vi "Begin.vi"(11 "Image Size":T1=enum."160x120") -> (0 "error out":errorcluster)   [LabVIEW 2011]
doc: "Called before other user functions, this VI is expected to open initial I/O refnums, load in file data, and do all program initialization. Notice that the <B>error out</B> terminal is simply used for data flow. Wiring it to other structures or subVIs ensures that this VI runs first."
uses:
  <vilib>/Rock Robotics/WPI/Camera/WPI_CameraImageSize.ctl
  <vilib>/Rock Robotics/SystemInterfaces/DIO/FPGA_DIOPWMChannel.ctl
  <vilib>/Rock Robotics/WPI/Joystick/WPI_JoystickDeviceEnum.ctl
  <vilib>/Rock Robotics/WPI/Camera/WPI_CameraWhite Balance Values.ctl
  <vilib>/Rock Robotics/WPI/Camera/WPI_CameraExposure Values.ctl
  <vilib>/Rock Robotics/WPI/Camera/WPI_CameraFrameRate.ctl
  <vilib>/Rock Robotics/SystemInterfaces/DIO/FPGA_DIOChannel.ctl
  <vilib>/Rock Robotics/WPI/Solenoid/WPI_SolenoidChannel.ctl
  <vilib>/Rock Robotics/SystemInterfaces/DIO/FPGA_DIORelayChannel.ctl
  <vilib>/Rock Robotics/SystemInterfaces/AI/FPGA_AIGyroChannel.ctl
  <vilib>/Rock Robotics/SystemInterfaces/Typedef/FPGA_TypedefDigitalModule.ctl
  <vilib>/Rock Robotics/WPI/Solenoid/WPI_SolenoidValue.ctl
  <vilib>/Rock Robotics/WPI/RobotDrive/WPI_RobotDriveOpen4MotorWithJaguar.vi
  <vilib>/Rock Robotics/WPI/Solenoid/WPI_SolenoidOpenDouble.vi
  <vilib>/Rock Robotics/WPI/Counter/WPI_CounterDigitalInputToDigitalSource.vi
  <vilib>/Rock Robotics/WPI/Counter/WPI_CounterOpen Gear Tooth Sensor Mode.vi
  <vilib>/Rock Robotics/WPI/MotorControl/WPI_MotorControlOpen Jaguar.vi
  <vilib>/Rock Robotics/WPI/Solenoid/WPI_SolenoidOpenSingle.vi
  <vilib>/Rock Robotics/WPI/Solenoid/WPI_SolenoidSetEnum.vi
  <vilib>/Rock Robotics/WPI/Counter/WPI_CounterOpen Semi Period Mode.vi
  <vilib>/Rock Robotics/WPI/MotorControl/WPI_MotorControlOpen Victor.vi
  <vilib>/Rock Robotics/WPI/Compressor/WPI_CompressorGetSetRefNum.vi
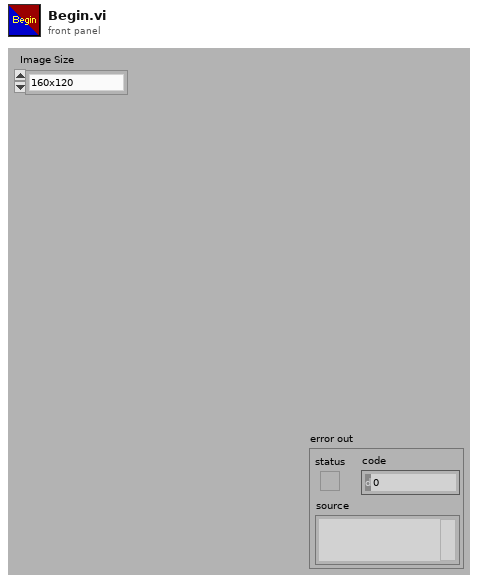
[diagram p1: front panel]
types:
  T1 = typedef "WPI_CameraImageSize.ctl" = enum16{"640x480", "320x240", "160x120"}
  T2 = typedef "FPGA_DIOPWMChannel.ctl" = enum8{"PWM 1", "PWM 2", "PWM 3", "PWM 4", "PWM 5", "PWM 6", "PWM 7", "PWM 8", "PWM 9", "PWM 10", "Invalid"}
  T3 = typedef "FPGA_DIOChannel.ctl" = enum8{"DIO 1", "DIO 2", "DIO 3", "DIO 4", "DIO 5", "DIO 6", "DIO 7", "DIO 8", "DIO 9", "DIO 10", "DIO 11", "DIO 12", "DIO 13", "DIO 14", "Invalid"}
  T4 = typedef "WPI_SolenoidValue.ctl" = enum16{"Off", "On", "Forward", "Reverse"}
  T5 = typedef "WPI_SolenoidChannel.ctl" = enum8{"Solenoid 1", "Solenoid 2", "Solenoid 3", "Solenoid 4", "Solenoid 5", "Solenoid 6", "Solenoid 7", "Solenoid 8", "Invalid"}
  T6 = typedef "WPI_JoystickDeviceEnum.ctl" = enum16{"USB 1", "USB 2", "USB 3", "USB 4", "Kinect 1", "Kinect 2"}
  T7 = typedef "FPGA_TypedefDigitalModule.ctl" = enum16{"Digital Module 1", "Digital Module 2"}
  T8 = typedef "FPGA_AIGyroChannel.ctl" = enum8{"AI 1", "AI 2", "Invalid"}
  T9 = typedef "FPGA_DIORelayChannel.ctl" = enum8{"Relay 1", "Relay 2", "Relay 3", "Relay 4", "Relay 5", "Relay 6", "Relay 7", "Relay 8", "Invalid"}
  T10 = typedef "WPI_CameraFrameRate.ctl" = u32
  T11 = typedef "WPI_CameraExposure Values.ctl" = enum16{"Auto", "Flicker-free 50 Hz", "Flicker-free 60 Hz", "Hold current"}
  T12 = typedef "WPI_CameraWhite Balance Values.ctl" = enum16{"Auto", "Fixed indoor", "Fixed outdoor 1", "Fixed outdoor 2", "Fixed fluorescent 1", "Fixed fluorescent 2", "Hold current"}
  T13 = typedef "WPI_RobotDriveDevRef.ctl" = cluster{"DevStatus":errorcluster, "Motors[]":T14[], "Square Inputs":bool, "Max Output":dbl, "Isochronous":bool}
  T14 = typedef "WPI_MotorControlDeviceRef.ctl" = cluster{"DeviceStatus":errorcluster, "Type":enum16{"PWM", "CAN"}, "PWM":cluster{"Digital Module":T7, "PWM Channel":T2, "DeadBand":T15}, "CAN":cluster{"Device Number":u8, "Control Mode":T16, "Semaphore":T17, "Max Vout":dbl}, "Invert":bool, "TransformRef":T18, "InvTransformRef":T18}
  T15 = typedef "WPI_PWMDeadband.ctl" = cluster{"Name":string, "maxPositivePwm":i32, "minPositivePwm":i32, "centerPwm":i32, "maxNegativePwm":i32, "minNegativePwm":i32, "angularRange":u16}
  T16 = typedef "WPI_CANJaguar_ControlMode.ctl" = enum8{"Percent VBus", "Current", "Speed", "Position", "Voltage"}
  T17 = typedef "Semaphore RefNum" = refnum<k1>
  T18 = typedef "WPI_PWMTransform_ConPane.ctl" = refnum<vi>
  T19 = typedef "WPI_JoystickDevRef.ctl" = cluster{"Device":T6}
  T20 = typedef "WPI_DigitalInputDevRef.ctl" = cluster{"DevStatus":errorcluster, "DIO Channel":T3, "Digital Module":T7}
  T21 = typedef "WPI_SolenoidDevRef.ctl" = cluster{"DevStatus":errorcluster, "Solenoid Module":T22, "Forward Solenoid Channel":T5, "Reverse Solenoid Channel":T5}
  T22 = typedef "FPGA_TypedefSolenoidModule.ctl" = enum16{"Solenoid Module 1", "Solenoid Module 2"}
  T23 = typedef "WPI_GyroDevRef.ctl" = cluster{"DevStatus":errorcluster, "Analog Module":T24, "Analog Channel":T25, "Offset":dbl, "Gain (VoltsPerDegree/Second)":dbl}
  T24 = typedef "FPGA_TypedefAnalogModule.ctl" = enum16{"Analog Module 1", "Analog Module 2"}
  T25 = typedef "FPGA_AIChannel.ctl" = enum8{"AI 1", "AI 2", "AI 3", "AI 4", "AI 5", "AI 6", "AI 7", "AI 8", "Invalid"}
  T26 = typedef "WPI_CompressorDevRef.ctl" = cluster{"DevStatus":errorcluster, "DigitalInputDevRef":T20, "RelayDevRef":T27}
  T27 = typedef "WPI_RelayDevRef.ctl" = cluster{"DevStatus":errorcluster, "Relay Channel":T9, "Digital Module":T7, "Relay Direction":T28}
  T28 = typedef "WPI_RelayDirection.ctl" = enum16{"Both directions", "Forward only", "Reverse only"}
  T29 = typedef "WPI_CameraDevRef.ctl" = cluster{"Camera Address":string, "CameraStatus":errorcluster, "Acquire Image Notifier":refnum<notifier>}
  T30 = typedef "FPGA_CounterEncoderSourceConvertionLVSourceType.ctl" = cluster{"DevStatus":errorcluster, "AnalogTriggerMode?":bool, "DigitalMode":cluster{"Digital Module":T7, "DIO Channel":T31}, "AnalogTriggerMode":cluster{"AnalogTriggerIndex":T32, "OutputType":T33}}
  T31 = typedef "FPGA_DIODigitalSourceChannel.ctl" = enum8{"DIO 1", "DIO 2", "DIO 3", "DIO 4", "DIO 5", "DIO 6", "DIO 7", "DIO 8", "DIO 9", "DIO 10", "DIO 11", "DIO 12", "DIO 13", "DIO 14", "Disabled"}
  T32 = typedef "FPGA_AnalogTriggerIndex.ctl" = enum8{"Trig 0", "Trig 1", "Trig 2", "Trig 3", "Trig 4", "Trig 5", "Trig 6", "Trig 7", "Invalid"}
  T33 = typedef "FPGA_AnalogTriggerOutType.ctl" = enum16{"InWindow", "TriggerState", "Rising", "Falling"}
  T34 = typedef "WPI_CounterDevRef.ctl" = cluster{"DevStatus":errorcluster, "CntIndex":T35}
  T35 = typedef "FPGA_CounterCtrSystemIndex.ctl" = enum8{"Ctr 0", "Ctr 1", "Ctr 2", "Ctr 3", "Ctr 4", "Ctr 5", "Ctr 6", "Ctr 7", "Invalid"}
  T36 = typedef "WPI_EncoderDevRef.ctl" = cluster{"DevStatus":errorcluster, "EncoderIndex":T37, "CounterIndex":T35, "DistancePerCount":dbl, "Decoding Type":T38}
  T37 = typedef "FPGA_EncoderIdx.ctl" = enum8{"Enc 0", "Enc 1", "Enc 2", "Enc 3", "Invalid"}
  T38 = typedef "WPI_EncoderType.ctl" = enum16{"1x", "2x", "4x"}
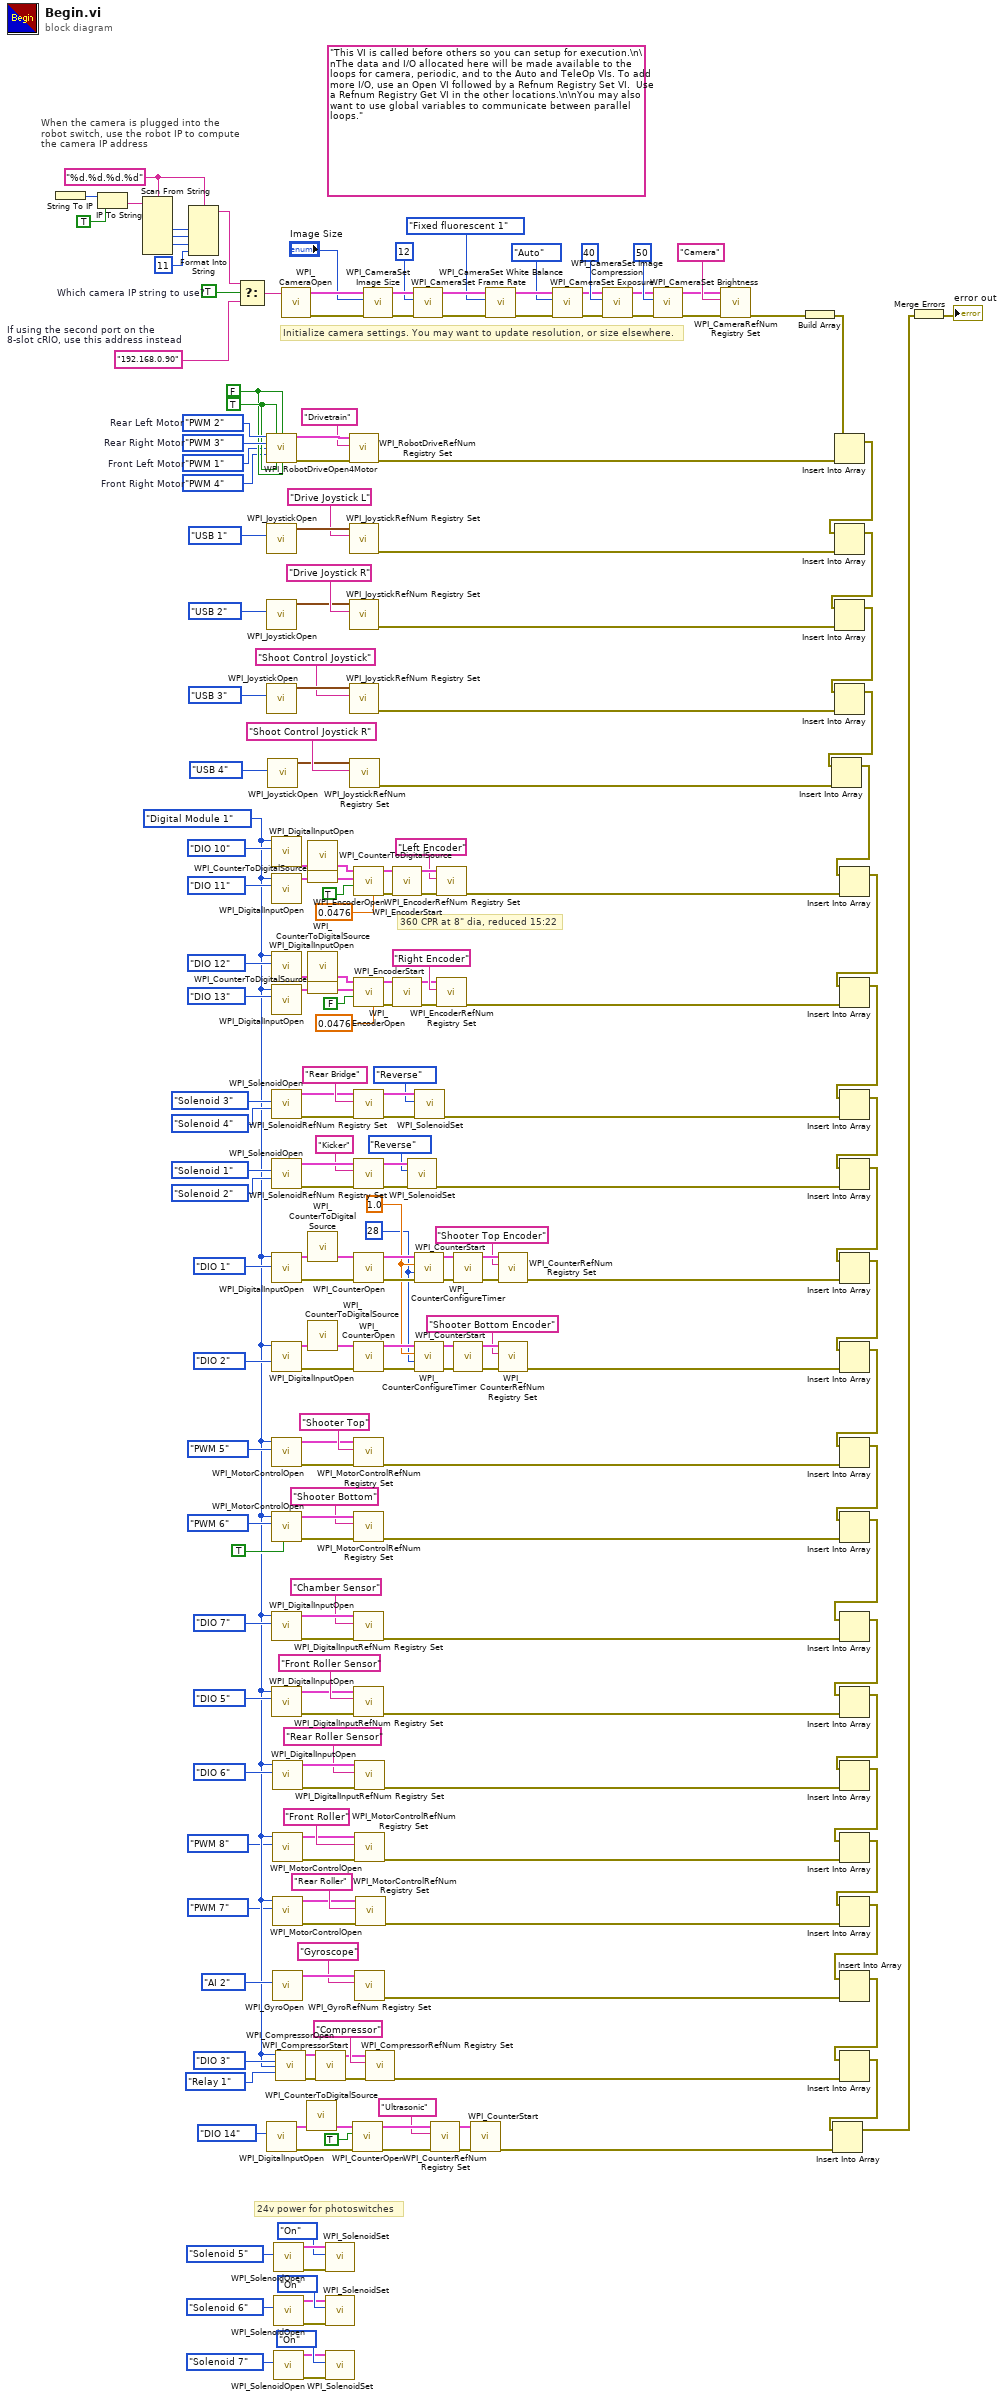
[diagram p0: block diagram]
diagram:
  w54 = u8 28 ("Number Samples to Average")
  w55 = 1.0 ("MaxPeriod (sec)")
  w26 = FPGA_TypedefDigitalModule."Digital Module 1" ("Relay Digital Module (Module 1)")
  w161 = FPGA_DIOPWMChannel."PWM 4"  # Front Right Motor
  w162 = FPGA_DIOPWMChannel."PWM 1"  # Front Left Motor
  w187 = TRUE  # Which camera IP string to use?
  w191 = "%d.%d.%d.%d" ("format string")
  (unwired) "This VI is called before others so you can setup for execution.\n\nThe data and I/O allocated here will be made available to the loops for camera, periodic, and to the Auto and TeleOp VIs. To add more I/O, use an Open VI followed by a Refnum Registry Set VI.  Use a Refnum Registry Get VI in the other locations.\n\nYou may also want to use global variables to communicate between parallel loops."
  w203 = FPGA_DIOPWMChannel."PWM 3"  # Rear Right Motor
  w204 = FPGA_DIOPWMChannel."PWM 2"  # Rear Left Motor
  w188 = "192.168.0.90"  # If using the second port on the 8-slot cRIO, use this address instead
  w164 = TRUE ("LeftMotorInverted")
  w163 = FALSE ("RightMotorInverted")
  # "24v power for photoswitches"
  # "360 CPR at 8\" dia, reduced 15:22"
  # "When the camera is plugged into the\nrobot switch, use the robot IP to compute\nthe camera IP address"
  # "Initialize camera settings. You may want to update resolution, or size elsewhere."
  n1 = String To IP() -> (0:w198:u32)  [unwired: 1 in]
  n2 = IP To String(1:TRUE ("dot notation? (F)"), 2:w198) -> (0:w196:string)
  n3 = Scan From String(format string=w191, input string=w196) -> (output 1=w195:i32, output 2=w194:i32, output 3=w193:i32)  [unwired: 7 in, 3 out]
  n4 = Format Into String(format string=w191, w195, w194, w193, 11 ("Compression")) -> (resulting string=w189:string)  [unwired: 2 in, 1 out]
  n5 = Select(t=w189, s=w187, f=w188) -> (s? t:f=w190:string)
  n6 = call-poly <vilib>:"WPI_RobotDriveOpen4Motor.vi"("Rear Left Motor"=w204, "Rear Left Motor Inverted"=w164, "Rear Right Motor Inverted"=w163, "Rear Right Motor"=w203, "Front Left Motor"=w162, "Front Right Motor"=w161, "Front Left Motor Inverted"=w164, "Front Right Motor Inverted"=w163) -> ("RobotDriveDevRef"=w226:T13, "error out"=w222:errorcluster)  [unwired: 6 in]
  n7 = call <vilib>:"WPI_JoystickOpen.vi"("JoystickDevice"=WPI_JoystickDeviceEnum."USB 1") -> ("JoystickDevRef"=w224:T19)  [unwired: 10 out]
  n8 = call <vilib>:"WPI_JoystickOpen.vi"("JoystickDevice"=WPI_JoystickDeviceEnum."USB 2") -> ("JoystickDevRef"=w158:T19)  [unwired: 10 out]
  n9 = call <vilib>:"WPI_JoystickOpen.vi"("JoystickDevice"=WPI_JoystickDeviceEnum."USB 3") -> ("JoystickDevRef"=w103:T19)  [unwired: 10 out]
  n10 = call <vilib>:"WPI_DigitalInputOpen.vi"("DIO Channel"=FPGA_DIOChannel."DIO 14") -> ("error out"=w14:errorcluster, "DigitalInputDevRef"=w15:T20)  [unwired: 9 in]
  n11 = call <vilib>:"WPI_JoystickOpen.vi"("JoystickDevice"=WPI_JoystickDeviceEnum."USB 4") -> ("JoystickDevRef"=w51:T19)  [unwired: 10 out]
  n12 = call <vilib>:"WPI_DigitalInputOpen.vi"("DIO Channel"=FPGA_DIOChannel."DIO 10", "Digital Module (Module 1)"=w26) -> ("DigitalInputDevRef"=w182:T20)  [unwired: 8 in, 1 out]
  n13 = call <vilib>:"WPI_DigitalInputOpen.vi"("DIO Channel"=FPGA_DIOChannel."DIO 11", "Digital Module (Module 1)"=w26) -> ("DigitalInputDevRef"=w181:T20)  [unwired: 8 in, 1 out]
  n14 = call <vilib>:"WPI_DigitalInputOpen.vi"("DIO Channel"=FPGA_DIOChannel."DIO 12", "Digital Module (Module 1)"=w26) -> ("DigitalInputDevRef"=w169:T20)  [unwired: 8 in, 1 out]
  n15 = call <vilib>:"WPI_DigitalInputOpen.vi"("DIO Channel"=FPGA_DIOChannel."DIO 13", "Digital Module (Module 1)"=w26) -> ("DigitalInputDevRef"=w170:T20)  [unwired: 8 in, 1 out]
  n16 = call-poly <vilib>:"WPI_SolenoidOpen.vi"("Reverse Solenoid Channel"=WPI_SolenoidChannel."Solenoid 4", "Forward Solenoid Channel"=WPI_SolenoidChannel."Solenoid 3") -> ("error out"=w125:errorcluster, "SolenoidDevRef"=w155:T21)  [unwired: 8 in]
  n17 = call-poly <vilib>:"WPI_SolenoidOpen.vi"("Reverse Solenoid Channel"=WPI_SolenoidChannel."Solenoid 2", "Forward Solenoid Channel"=WPI_SolenoidChannel."Solenoid 1") -> ("error out"=w124:errorcluster, "SolenoidDevRef"=w129:T21)  [unwired: 8 in]
  n18 = call <vilib>:"WPI_DigitalInputOpen.vi"("DIO Channel"=FPGA_DIOChannel."DIO 1", "Digital Module (Module 1)"=w26) -> ("error out"=w150:errorcluster, "DigitalInputDevRef"=w152:T20)  [unwired: 8 in]
  n19 = call <vilib>:"WPI_DigitalInputOpen.vi"("DIO Channel"=FPGA_DIOChannel."DIO 2", "Digital Module (Module 1)"=w26) -> ("error out"=w144:errorcluster, "DigitalInputDevRef"=w146:T20)  [unwired: 8 in]
  n20 = call-poly <vilib>:"WPI_MotorControlOpen.vi"("PWM Channel"=FPGA_DIOPWMChannel."PWM 5", "Digital Module (Module 1)"=w26) -> ("error out"=w136:errorcluster, "MotorControlDeviceRef"=w137:T14)  [unwired: 8 in]
  n21 = call-poly <vilib>:"WPI_MotorControlOpen.vi"("Invert"=TRUE, "PWM Channel"=FPGA_DIOPWMChannel."PWM 6", "Digital Module (Module 1)"=w26) -> ("error out"=w134:errorcluster, "MotorControlDeviceRef"=w133:T14)  [unwired: 7 in]
  n22 = call <vilib>:"WPI_DigitalInputOpen.vi"("DIO Channel"=FPGA_DIOChannel."DIO 7", "Digital Module (Module 1)"=w26) -> ("error out"=w93:errorcluster, "DigitalInputDevRef"=w97:T20)  [unwired: 8 in]
  n23 = call <vilib>:"WPI_DigitalInputOpen.vi"("DIO Channel"=FPGA_DIOChannel."DIO 5", "Digital Module (Module 1)"=w26) -> ("error out"=w92:errorcluster, "DigitalInputDevRef"=w90:T20)  [unwired: 8 in]
  n24 = call <vilib>:"WPI_DigitalInputOpen.vi"("DIO Channel"=FPGA_DIOChannel."DIO 6", "Digital Module (Module 1)"=w26) -> ("error out"=w85:errorcluster, "DigitalInputDevRef"=w87:T20)  [unwired: 8 in]
  n25 = call-poly <vilib>:"WPI_MotorControlOpen.vi"("PWM Channel"=FPGA_DIOPWMChannel."PWM 8", "Digital Module (Module 1)"=w26) -> ("error out"=w80:errorcluster, "MotorControlDeviceRef"=w3:T14)  [unwired: 8 in]
  n26 = call-poly <vilib>:"WPI_MotorControlOpen.vi"("PWM Channel"=FPGA_DIOPWMChannel."PWM 7", "Digital Module (Module 1)"=w26) -> ("error out"=w25:errorcluster, "MotorControlDeviceRef"=w2:T14)  [unwired: 8 in]
  n27 = call <vilib>:"WPI_GyroOpen.vi"("Analog Channel"=FPGA_AIGyroChannel."AI 2") -> ("GyroDevRef"=w76:T23)  [unwired: 8 in, 2 out]
  n28 = call-poly <vilib>:"WPI_SolenoidOpen.vi"("Solenoid Channel"=WPI_SolenoidChannel."Solenoid 5") -> ("error out"=w46:errorcluster, "SolenoidDevRef"=w45:T21)  [unwired: 9 in]
  n29 = call-poly <vilib>:"WPI_SolenoidOpen.vi"("Solenoid Channel"=WPI_SolenoidChannel."Solenoid 6") -> ("error out"=w41:errorcluster, "SolenoidDevRef"=w42:T21)  [unwired: 9 in]
  n30 = call-poly <vilib>:"WPI_SolenoidOpen.vi"("Solenoid Channel"=WPI_SolenoidChannel."Solenoid 7") -> ("error out"=w1:errorcluster, "SolenoidDevRef"=w20:T21)  [unwired: 9 in]
  n31 = call <vilib>:"WPI_CompressorOpen.vi"("Pressure Switch Digital Module (Module 1)"=w26, "Pressure Switch DIO Channel"=FPGA_DIOChannel."DIO 3", "Relay Digital Module (Module 1)"=w26, "Relay Channel"=FPGA_DIORelayChannel."Relay 1") -> ("CompressorDevRef"=w67:T26, "error out"=w65:errorcluster)  [unwired: 10 in]
  n32 = call <vilib>:"WPI_CameraOpen.vi"("Camera Address"=w190) -> ("error out"=w213:errorcluster, "CameraDevRef"=w214:T29)  [unwired: 1 in, 8 out]
  n33 = call-poly <vilib>:"WPI_CounterToDigitalSource.vi"("DigitalInputDevRef"=w15) -> ("Digital Source"=w17:T30)  [unwired: 6 in]
  n34 = call-poly <vilib>:"WPI_CounterToDigitalSource.vi"("DigitalInputDevRef"=w182) -> ("Digital Source"=w184:T30)  [unwired: 6 in]
  n35 = call-poly <vilib>:"WPI_CounterToDigitalSource.vi"("DigitalInputDevRef"=w181) -> ("Digital Source"=w183:T30)  [unwired: 6 in]
  n36 = call-poly <vilib>:"WPI_CounterToDigitalSource.vi"("DigitalInputDevRef"=w169) -> ("Digital Source"=w167:T30)  [unwired: 6 in]
  n37 = call-poly <vilib>:"WPI_CounterToDigitalSource.vi"("DigitalInputDevRef"=w170) -> ("Digital Source"=w168:T30)  [unwired: 6 in]
  n38 = call-poly <vilib>:"WPI_CounterToDigitalSource.vi"("DigitalInputDevRef"=w152) -> ("Digital Source"=w151:T30)  [unwired: 6 in]
  n39 = call-poly <vilib>:"WPI_CounterToDigitalSource.vi"("DigitalInputDevRef"=w146) -> ("Digital Source"=w145:T30)  [unwired: 6 in]
  n40 = call <vilib>:"WPI_CompressorStart.vi"("error in (no error)"=w65, "CompressorDevRef"=w67) -> ("error out"=w64:errorcluster, "CompressorDevRef"=w66:T26)  [unwired: 8 in]
  n41 = call-poly <vilib>:"WPI_SolenoidSet.vi"("error in (no error)"=w46, "Value"=WPI_SolenoidValue."On", "SolenoidDevRef"=w45) -> ()  [unwired: 7 in, 2 out]
  n42 = call-poly <vilib>:"WPI_SolenoidSet.vi"("error in (no error)"=w41, "Value"=WPI_SolenoidValue."On", "SolenoidDevRef"=w42) -> ()  [unwired: 7 in, 2 out]
  n43 = call-poly <vilib>:"WPI_SolenoidSet.vi"("error in (no error)"=w1, "Value"=WPI_SolenoidValue."On", "SolenoidDevRef"=w20) -> ()  [unwired: 7 in, 2 out]
  n44 = call <vilib>:"WPI_RobotDriveRefNum Registry Set.vi"("error in (no error)"=w222, "refnum name"="Drivetrain", "RobotDriveDevRef"=w226) -> ("error out"=w121:errorcluster)  [unwired: 8 out]
  n45 = call <vilib>:"WPI_JoystickRefNum Registry Set.vi"("refnum name"="Drive Joystick L", "JoystickDevRef"=w224) -> ("error out"=w119:errorcluster)  [unwired: 1 in, 8 out]
  n46 = call <vilib>:"WPI_JoystickRefNum Registry Set.vi"("refnum name"="Drive Joystick R", "JoystickDevRef"=w158) -> ("error out"=w112:errorcluster)  [unwired: 1 in, 8 out]
  n47 = call <vilib>:"WPI_JoystickRefNum Registry Set.vi"("refnum name"="Shoot Control Joystick", "JoystickDevRef"=w103) -> ("error out"=w100:errorcluster)  [unwired: 1 in, 8 out]
  n48 = call <vilib>:"WPI_JoystickRefNum Registry Set.vi"("refnum name"="Shoot Control Joystick R", "JoystickDevRef"=w51) -> ("error out"=w50:errorcluster)  [unwired: 1 in, 8 out]
  n49 = call-poly <vilib>:"WPI_CounterOpen.vi"("error in (no error)"=w14, "High Pulse (T)"=TRUE, "Source"=w17) -> ("error out"=w12:errorcluster, "CounterDevRef"=w13:T34)  [unwired: 7 in]
  n50 = call <vilib>:"WPI_EncoderOpen.vi"("DistancePerCount"=0.0476, "Invert Direction (False)"=TRUE, "BSource"=w183, "ASource"=w184) -> ("error out"=w185:errorcluster, "EncoderDevRef"=w186:T36)  [unwired: 6 in]
  n51 = call <vilib>:"WPI_EncoderOpen.vi"("DistancePerCount"=0.0476, "Invert Direction (False)"=FALSE, "BSource"=w168, "ASource"=w167) -> ("error out"=w166:errorcluster, "EncoderDevRef"=w165:T36)  [unwired: 6 in]
  n52 = call <vilib>:"WPI_SolenoidRefNum Registry Set.vi"("error in (no error)"=w125, "refnum name"="Rear Bridge", "SolenoidDevRef"=w155) -> ("error out"=w37:errorcluster, "SolenoidDevRef"=w39:T21)  [unwired: 7 in]
  n53 = call <vilib>:"WPI_SolenoidRefNum Registry Set.vi"("error in (no error)"=w124, "refnum name"="Kicker", "SolenoidDevRef"=w129) -> ("error out"=w35:errorcluster, "SolenoidDevRef"=w34:T21)  [unwired: 7 in]
  n54 = call-poly <vilib>:"WPI_CounterOpen.vi"("error in (no error)"=w150, "Source"=w151) -> ("error out"=w63:errorcluster, "CounterDevRef"=w62:T34)  [unwired: 8 in]
  n55 = call-poly <vilib>:"WPI_CounterOpen.vi"("error in (no error)"=w144, "Source"=w145) -> ("error out"=w56:errorcluster, "CounterDevRef"=w57:T34)  [unwired: 8 in]
  n56 = call <vilib>:"WPI_MotorControlRefNum Registry Set.vi"("error in (no error)"=w136, "refnum name"="Shooter Top", "MotorControlDevRef"=w137) -> ("error out"=w107:errorcluster)  [unwired: 7 in, 1 out]
  n57 = call <vilib>:"WPI_MotorControlRefNum Registry Set.vi"("error in (no error)"=w134, "refnum name"="Shooter Bottom", "MotorControlDevRef"=w133) -> ("error out"=w105:errorcluster)  [unwired: 7 in, 1 out]
  n58 = call <vilib>:"WPI_DigitalInputRefNum Registry Set.vi"("error in (no error)"=w93, "refnum name"="Chamber Sensor", "DigitalInputDevRef"=w97) -> ("error out"=w95:errorcluster)  [unwired: 7 in, 1 out]
  n59 = call <vilib>:"WPI_DigitalInputRefNum Registry Set.vi"("error in (no error)"=w92, "refnum name"="Front Roller Sensor", "DigitalInputDevRef"=w90) -> ("error out"=w84:errorcluster)  [unwired: 7 in, 1 out]
  n60 = call <vilib>:"WPI_DigitalInputRefNum Registry Set.vi"("error in (no error)"=w85, "refnum name"="Rear Roller Sensor", "DigitalInputDevRef"=w87) -> ("error out"=w82:errorcluster)  [unwired: 7 in, 1 out]
  n61 = call <vilib>:"WPI_MotorControlRefNum Registry Set.vi"("error in (no error)"=w80, "refnum name"="Front Roller", "MotorControlDevRef"=w3) -> ("error out"=w79:errorcluster)  [unwired: 7 in, 1 out]
  n62 = call <vilib>:"WPI_GyroRefNum Registry Set.vi"("refnum name"="Gyroscope", "GyroDevRef"=w76) -> ("error out"=w74:errorcluster)  [unwired: 8 in, 1 out]
  n63 = call <vilib>:"WPI_MotorControlRefNum Registry Set.vi"("error in (no error)"=w25, "refnum name"="Rear Roller", "MotorControlDevRef"=w2) -> ("error out"=w24:errorcluster)  [unwired: 7 in, 1 out]
  n64 = call <vilib>:"WPI_CameraSet Image Size.vi"("error in (no error)"=w213, "Image Size"="Image Size", "CameraDevRef"=w214) -> ("error out"=w212:errorcluster, "CameraDevRef Out"=w215:T29)  [unwired: 7 out]
  n65 = call <vilib>:"WPI_CompressorRefNum Registry Set.vi"("error in (no error)"=w64, "refnum name"="Compressor", "CompressorDevRef"=w66) -> ("error out"=w73:errorcluster)  [unwired: 7 in, 1 out]
  n66 = call <vilib>:"WPI_EncoderStart.vi"("error in (no error)"=w185, "EncoderDevRef"=w186) -> ("error out"=w178:errorcluster, "EncoderDevRef"=w177:T36)  [unwired: 8 in]
  n67 = call <vilib>:"WPI_EncoderStart.vi"("error in (no error)"=w166, "EncoderDevRef"=w165) -> ("error out"=w173:errorcluster, "EncoderDevRef"=w174:T36)  [unwired: 8 in]
  n68 = call-poly <vilib>:"WPI_SolenoidSet.vi"("error in (no error)"=w35, "Value"=WPI_SolenoidValue."Reverse", "SolenoidDevRef"=w34) -> ("error out"=w32:errorcluster)  [unwired: 7 in, 1 out]
  n69 = call <vilib>:"WPI_CameraSet Frame Rate.vi"("error in (no error)"=w212, "Frame Rate (fps)"=T10 12, "CameraDevRef"=w215) -> ("error out"=w211:errorcluster, "CameraDevRef Out"=w217:T29)  [unwired: 7 out]
  n70 = call <vilib>:"WPI_CounterConfigureTimer.vi"("error in (no error)"=w63, "Number Samples to Average"=w54, "MaxPeriod (sec)"=w55, "CounterDevRef in"=w62) -> ("error out"=w60:errorcluster, "CounterDevRef out"=w61:T34)  [unwired: 6 in]
  n71 = call <vilib>:"WPI_CounterConfigureTimer.vi"("error in (no error)"=w56, "Number Samples to Average"=w54, "MaxPeriod (sec)"=w55, "CounterDevRef in"=w57) -> ("error out"=w59:errorcluster, "CounterDevRef out"=w58:T34)  [unwired: 6 in]
  n72 = call-poly <vilib>:"WPI_SolenoidSet.vi"("error in (no error)"=w37, "Value"=WPI_SolenoidValue."Reverse", "SolenoidDevRef"=w39) -> ("error out"=w36:errorcluster)  [unwired: 7 in, 1 out]
  n73 = call <vilib>:"WPI_CounterRefNum Registry Set.vi"("error in (no error)"=w12, "refnum name"="Ultrasonic", "CounterDevRef"=w13) -> ("error out"=w10:errorcluster, "CounterDevRef"=w11:T34)  [unwired: 7 in]
  n74 = call <vilib>:"WPI_EncoderRefNum Registry Set.vi"("error in (no error)"=w178, "refnum name"="Left Encoder", "EncoderDevRef"=w177) -> ("error out"=w118:errorcluster)  [unwired: 7 in, 1 out]
  n75 = call <vilib>:"WPI_EncoderRefNum Registry Set.vi"("error in (no error)"=w173, "refnum name"="Right Encoder", "EncoderDevRef"=w174) -> ("error out"=w116:errorcluster)  [unwired: 7 in, 1 out]
  n76 = call <vilib>:"WPI_CounterStart.vi"("error in (no error)"=w60, "CounterDevRef in"=w61) -> ("error out"=w149:errorcluster, "CounterDevRef out"=w148:T34)  [unwired: 8 in]
  n77 = call <vilib>:"WPI_CounterStart.vi"("error in (no error)"=w59, "CounterDevRef in"=w58) -> ("error out"=w143:errorcluster, "CounterDevRef out"=w142:T34)  [unwired: 8 in]
  n78 = call <vilib>:"WPI_CounterStart.vi"("error in (no error)"=w10, "CounterDevRef in"=w11) -> ("error out"=w8:errorcluster)  [unwired: 8 in, 1 out]
  n79 = call <vilib>:"WPI_CameraSet White Balance.vi"("error in (no error)"=w211, "White Balance"=WPI_CameraWhite_Balance_Values."Fixed fluorescent 1", "CameraDevRef"=w217) -> ("error out"=w210:errorcluster, "CameraDevRef Out"=w216:T29)  [unwired: 7 out]
  n80 = call <vilib>:"WPI_CounterRefNum Registry Set.vi"("error in (no error)"=w149, "refnum name"="Shooter Top Encoder", "CounterDevRef"=w148) -> ("error out"=w111:errorcluster)  [unwired: 7 in, 1 out]
  n81 = call <vilib>:"WPI_CounterRefNum Registry Set.vi"("error in (no error)"=w143, "refnum name"="Shooter Bottom Encoder", "CounterDevRef"=w142) -> ("error out"=w109:errorcluster)  [unwired: 7 in, 1 out]
  n82 = call <vilib>:"WPI_CameraSet Exposure.vi"("error in (no error)"=w210, "Exposure"=WPI_CameraExposure_Values."Auto", "CameraDevRef"=w216) -> ("error out"=w209:errorcluster, "CameraDevRef Out"=w219:T29)  [unwired: 7 out]
  n83 = call <vilib>:"WPI_CameraSet Image Compression.vi"("error in (no error)"=w209, "Compression"=40, "CameraDevRef"=w219) -> ("error out"=w208:errorcluster, "CameraDevRef Out"=w218:T29)  [unwired: 7 out]
  n84 = call <vilib>:"WPI_CameraSet Brightness.vi"("error in (no error)"=w208, "Brightness"=50, "CameraDevRef"=w218) -> ("error out"=w206:errorcluster, "CameraDevRef Out"=w207:T29)  [unwired: 7 out]
  n85 = call <vilib>:"WPI_CameraRefNum Registry Set.vi"("error in (no error)"=w206, "refnum name"="Camera", "CameraDevRef"=w207) -> ("error out"=w123:errorcluster)  [unwired: 8 out]
  n86 = Build Array(w123) -> (w122:errorcluster[])
  n87 = Insert Into Array(array=w122, new element=w121) -> (w120:errorcluster[])  [unwired: 1 in]
  n88 = Insert Into Array(array=w120, new element=w119) -> (w113:errorcluster[])  [unwired: 1 in]
  n89 = Insert Into Array(array=w113, new element=w112) -> (w99:errorcluster[])  [unwired: 1 in]
  n90 = Insert Into Array(array=w99, new element=w100) -> (w49:errorcluster[])  [unwired: 1 in]
  n91 = Insert Into Array(array=w49, new element=w50) -> (w48:errorcluster[])  [unwired: 1 in]
  n92 = Insert Into Array(array=w48, new element=w118) -> (w117:errorcluster[])  [unwired: 1 in]
  n93 = Insert Into Array(array=w117, new element=w116) -> (w115:errorcluster[])  [unwired: 1 in]
  n94 = Insert Into Array(array=w115, new element=w36) -> (w114:errorcluster[])  [unwired: 1 in]
  n95 = Insert Into Array(array=w114, new element=w32) -> (w110:errorcluster[])  [unwired: 1 in]
  n96 = Insert Into Array(array=w110, new element=w111) -> (w108:errorcluster[])  [unwired: 1 in]
  n97 = Insert Into Array(array=w108, new element=w109) -> (w106:errorcluster[])  [unwired: 1 in]
  n98 = Insert Into Array(array=w106, new element=w107) -> (w104:errorcluster[])  [unwired: 1 in]
  n99 = Insert Into Array(array=w104, new element=w105) -> (w94:errorcluster[])  [unwired: 1 in]
  n100 = Insert Into Array(array=w94, new element=w95) -> (w83:errorcluster[])  [unwired: 1 in]
  n101 = Insert Into Array(array=w83, new element=w84) -> (w81:errorcluster[])  [unwired: 1 in]
  n102 = Insert Into Array(array=w81, new element=w82) -> (w78:errorcluster[])  [unwired: 1 in]
  n103 = Insert Into Array(array=w78, new element=w79) -> (w23:errorcluster[])  [unwired: 1 in]
  n104 = Insert Into Array(array=w23, new element=w24) -> (w22:errorcluster[])  [unwired: 1 in]
  n105 = Insert Into Array(array=w22, new element=w74) -> (w71:errorcluster[])  [unwired: 1 in]
  n106 = Insert Into Array(array=w71, new element=w73) -> (w6:errorcluster[])  [unwired: 1 in]
  n107 = Insert Into Array(array=w6, new element=w8) -> (w7:errorcluster[])  [unwired: 1 in]
  n108 = Merge Errors(w7) -> (→"error out":errorcluster)
